vi "MM9.UnloadObjs.vi"(0 "i ref in":refnum<vi>, 2 "ObjsToUnload":string[](array[string]), 5 "error in (no error)":errorcluster) -> (14 "i ref out":refnum<vi>, 19 "error out":errorcluster)   [LabVIEW 2014, in "MM9.lvlib"]
doc: "Unloads all objects specified."
uses:
  MM9.lvlib
  CS_Core/CSSystem/CoreLib/CoreLib.string 2 byte array.vi
  CS_Core/CSSystem/CoreLib/CoreLib.lvlib
  CS_Core/BaseProcess/BaseProcess.lvlib
  CS_Core/CSSystem/CSSystemLib/CSSystemLib.lvlib
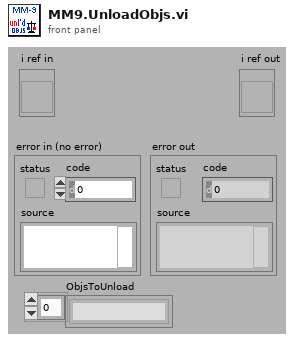
[diagram p1: front panel]
types:
  T1 = typedef "CoreDefs.rawDataType.ctl" = i8[]
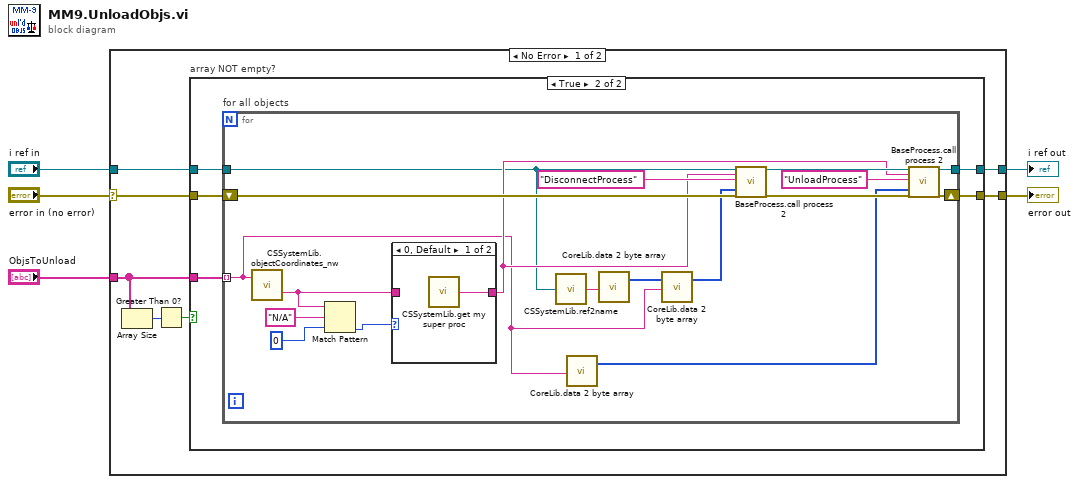
[diagram p0: block diagram]
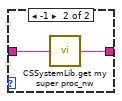
[diagram p3: hidden frame]
diagram:
  n1 = case shown="No Error" "error in (no error)" {
    selector: "error in (no error)" -> [w6 w41]
    tunnel: [w12 w42] -> w5
    tunnel: [w11 w41] -> w4
    tunnel: "ObjsToUnload" -> [w8 _]
    tunnel: "i ref in" -> [w7 w42]
    frame No Error {
      n2 = Array Size(array=w8) -> (size(s)=w10:i32)
      n3 = Greater Than 0?(x=w10) -> (x > 0?=w9:bool)
      n4 = case "array NOT empty?" shown="True" w9 {
        tunnel: w8 -> [_ w19]
        tunnel: w7 -> [w14 w18]
        tunnel: w6 -> [w13 w17]
        tunnel: [w14 w16] -> w12
        tunnel: [w13 w15] -> w11
        frame False {
        }
        frame True {
          n5 = for "for all objects" {
            tunnel: w19 -> [w20] mode=indexing
            tunnel: [w37] -> w16
            shift-right: [w36] -> w15
            shift-left: w17 -> [w33]
            tunnel: w18 -> [w24]
            n6 = call "CSSystemLib.objectCoordinates_nw.vi"("name"=w20) -> ("systemID"=w28:string)  [unwired: 15 in, 3 out]
            n7 = Match Pattern(string=w28, regular expression="N/A", offset (0)=0) -> (offset past match=w25:i32)  [unwired: 3 out]
            n8 = case shown="0, Default" w25 {
              tunnel: [w38 w40] -> w31
              tunnel: w28 -> [_ w39]
              frame 0, Default {
                n9 = call "CSSystemLib.get my super proc.vi"() -> ("name"=w38:string)  [unwired: 1 in]
              }
              frame -1 {
                n10 = call "CSSystemLib.get my super proc_nw.vi"("systemID"=w39) -> ("superProcName"=w40:string)
              }
            }
            n11 = call "CSSystemLib.ref2name.vi"("obj refnum"=w24) -> ("name"=w23:string)
            n12 = call-poly "CoreLib.data 2 byte array.vi"("string"=w20) -> ("byteArray out"=w29:T1)  [unwired: 18 in]
            n13 = call-poly "CoreLib.data 2 byte array.vi"("string"=w23) -> ("byteArray out"=w22:T1)  [unwired: 18 in]
            n14 = call-poly "CoreLib.data 2 byte array.vi"("byteArray"=w22, "string"=w20) -> ("byteArray out"=w21:T1)  [unwired: 17 in]
            n15 = call "BaseProcess.call process 2.vi"("i ref in"=w24, "Object"=w31, "Selector"="DisconnectProcess", "Data"=w21, "error in (no error)"=w33) -> ("i ref out"=w35:refnum<vi>, "error out"=w34:errorcluster)  [unwired: 13 in]
            n16 = call "BaseProcess.call process 2.vi"("i ref in"=w35, "Object"=w31, "Selector"="UnloadProcess", "Data"=w29, "error in (no error)"=w34) -> ("i ref out"=w37:refnum<vi>, "error out"=w36:errorcluster)  [unwired: 13 in]
          }
        }
      }
    }
    frame Error {
    }
  }
  "error out" <- w4
  "i ref out" <- w5
